vi "Check_for_Do.vi"(8 "error in (no error)":errorcluster, 11 "VI ref":refnum<vi>) -> (0 "error out":errorcluster, 1 "Do.vi Ref":refnum<vi>, 2 "Has Do.vi?":bool, 3 "VI ref out":refnum<vi>)   [LabVIEW 2015]
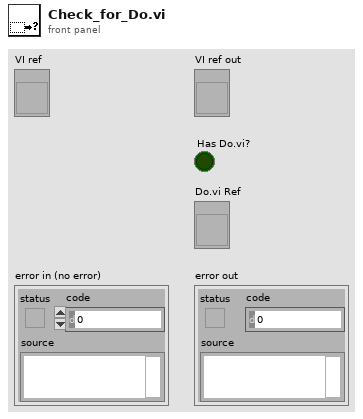
[diagram p1: front panel]
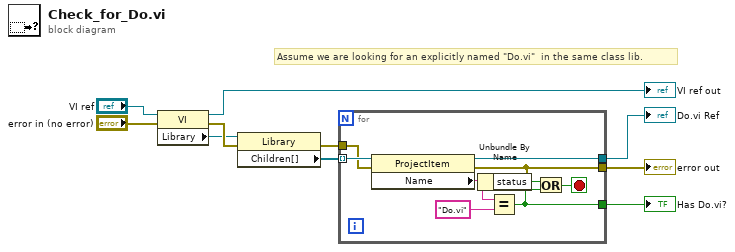
[diagram p0: block diagram]
diagram:
  # "Assume we are looking for an explicitly named \"Do.vi\"  in the same class lib."
  n1 = property class="VI"(reference="VI ref", error in="error in (no error)") -> (reference out=→"VI ref out":refnum<vi>, error out=w10:errorcluster, "Library"=w9:refnum<vi>)
  n2 = property class="Library"(reference=w9, error in=w10) -> (error out=w7:errorcluster, "Children[]"=w8:refnum<vi>[])  [unwired: 1 out]
  n3 = for {
    tunnel: w8 -> [w19] mode=indexing
    tunnel: [w15] -> w4
    tunnel: w7 -> [w16]
    tunnel: [w13] -> w3
    tunnel: [w12] -> w2
    stop <- w14 stop-if-true
    n4 = property class="ProjectItem"(reference=w19, error in=w16) -> (reference out=w13:refnum<vi>, error out=w12:errorcluster, "Name"=w17:string)
    n5 = Unbundle By Name(w12) -> ("status"=w11:bool)
    n6 = Equal?(x=w17, y="Do.vi") -> (x = y?=w15:bool)
    n7 = Or(x=w11, y=w15) -> (x .or. y?=w14:bool)
  }
  "Has Do.vi?" <- w4
  "error out" <- w2
  "Do.vi Ref" <- w3
